vi "KikusuiCode.vi"() -> ()   [LabVIEW 2020]
panel:
  out "Error Code":dbl
  in  "Command String":string
  out "return count":u32
  out "read buffer":string
  out "error out":errorcluster
  in  "VISA resource name":refnum<visa-resource-name>
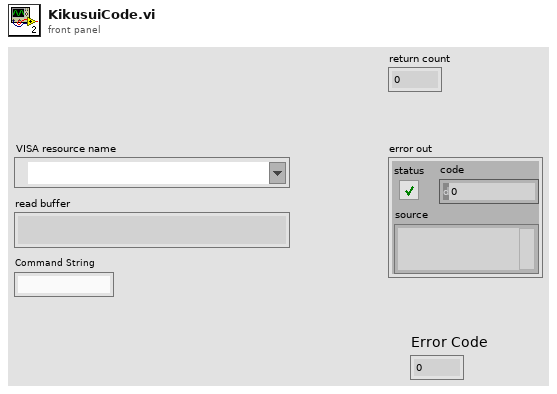
[diagram p1: front panel]
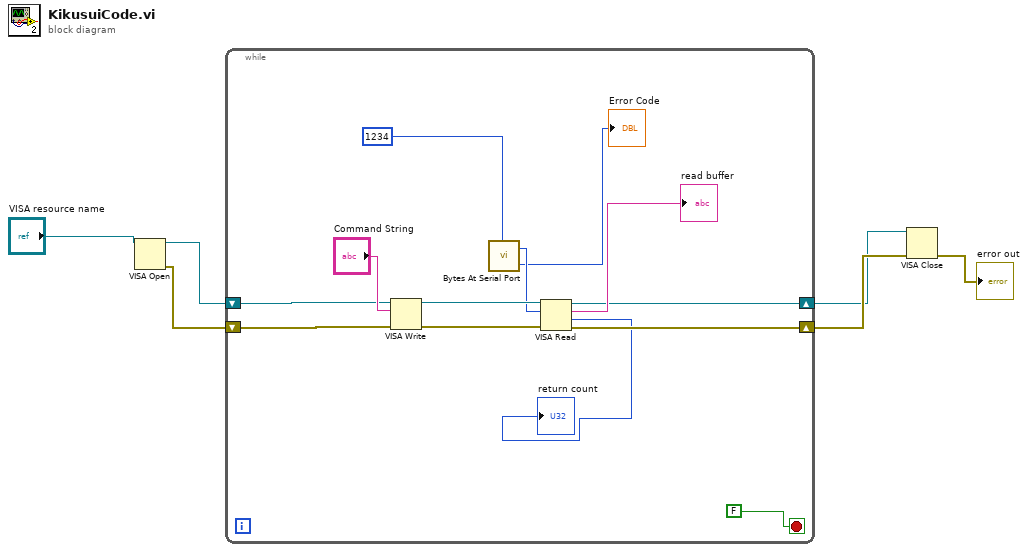
[diagram p0: block diagram]
diagram:
  n1 = VISA Open(VISA resource name="VISA resource name") -> (VISA resource name=w3:refnum<visa-resource-name>, error out=w4:errorcluster)  [unwired: 4 in]
  n2 = while {
    shift-right: [w13] -> w2
    shift-left: w4 -> [w15]
    shift-right: [w12] -> w1
    shift-left: w3 -> [w14]
    stop <- FALSE ("stop") stop-if-true
    n3 = VISA Write(VISA resource name=w14, write buffer="Command String", error in (no error)=w15) -> (VISA resource name out=w17:refnum<visa-resource-name>, error out=w18:errorcluster)  [unwired: 1 out]
    n4 = call <vilib>:"Bytes At Serial Port.vi"("port number"=1234) -> ("byte count"=w9:u32, "error code"=→"Error Code":i32)
    n5 = VISA Read(VISA resource name=w17, byte count=w9, error in (no error)=w18) -> (VISA resource name out=w12:refnum<visa-resource-name>, read buffer=→"read buffer":string, return count=→"return count":u32, error out=w13:errorcluster)
  }
  n6 = VISA Close(VISA resource name=w1, error in (no error)=w2) -> (error out=→"error out":errorcluster)
